vi "Create Timing Diagram from Trigger Position.vi"(11 "Relative Trigger Position in":dbl[](array[numeric])) -> (3 "Timing Diagram":digitalwaveform[](array[waveform]))   [LabVIEW 2024]
uses:
  <vilib>/Waveform/DWDTOps.llb/Digital Pattern Generator (Single Value).vi
  <vilib>/Waveform/DWDTOps.llb/DWDT Append Digital Samples.vi
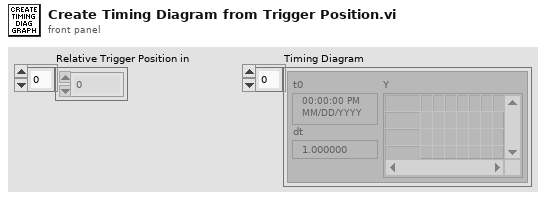
[diagram p1: front panel]
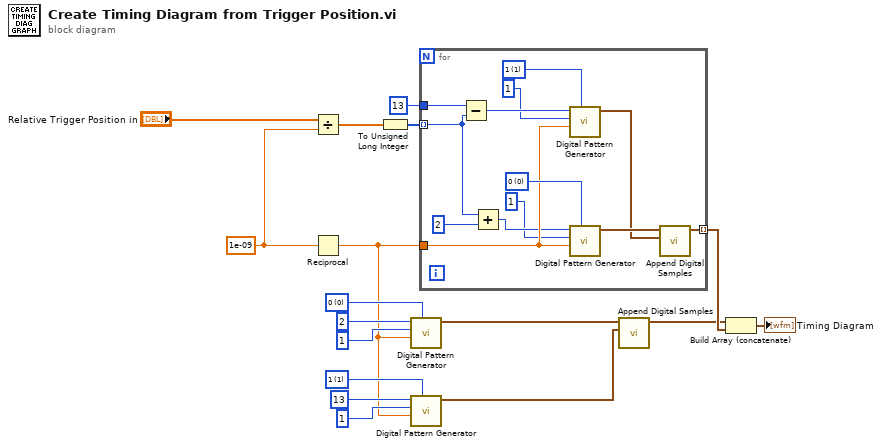
[diagram p0: block diagram]
diagram:
  w7 = u8 1 items=["0", "1", "Z", "L", "H", "X", "T", "V"] ("value")
  w10 = u8 0 items=["0", "1", "Z", "L", "H", "X", "T", "V"] ("value")
  w16 = 1e-09 ("y")
  n1 = Divide(x="Relative Trigger Position in", y=w16) -> (x/y=w2:dbl[])
  n2 = Reciprocal(x=w16) -> (1/x=w1:dbl)
  n3 = To Unsigned Long Integer(number=w2) -> (unsigned 32bit integer=w3:u32[])
  n4 = call-poly <vilib>:"Digital Pattern Generator.vi"("value"=w10, "sample rate"=w1, "number of signals"=u32 1, "number of samples"=u32 2) -> ("digital waveform"=w6:digitalwaveform)  [unwired: 6 in, 1 out]
  n5 = call-poly <vilib>:"Digital Pattern Generator.vi"("value"=w7, "sample rate"=w1, "number of signals"=u32 1, "number of samples"=u32 13) -> ("digital waveform"=w5:digitalwaveform)  [unwired: 6 in, 1 out]
  n6 = for {
    tunnel: w3 -> [w21] mode=indexing
    tunnel: u32 13 -> [w30]
    tunnel: [w26] -> w14 mode=indexing
    tunnel: w1 -> [w25]
    w29 = u8 0 items=["0", "1", "Z", "L", "H", "X", "T", "V"] ("value")
    w28 = u8 1 items=["0", "1", "Z", "L", "H", "X", "T", "V"] ("value")
    n7 = Subtract(x=w30, y=w21) -> (x-y=w20:u32)
    n8 = Add(x=w21, y=u32 2) -> (x+y=w22:u32)
    n9 = call-poly <vilib>:"Digital Pattern Generator.vi"("value"=w28, "sample rate"=w25, "number of signals"=u32 1, "number of samples"=w20) -> ("digital waveform"=w23:digitalwaveform)  [unwired: 6 in, 1 out]
    n10 = call-poly <vilib>:"Digital Pattern Generator.vi"("value"=w29, "sample rate"=w25, "number of signals"=u32 1, "number of samples"=w22) -> ("digital waveform"=w24:digitalwaveform)  [unwired: 6 in, 1 out]
    n11 = call-poly <vilib>:"Append Digital Samples.vi"("digital waveform B"=w23, "digital waveform A"=w24) -> ("digital waveform out"=w26:digitalwaveform)  [unwired: 8 in, 1 out]
  }
  n12 = call-poly <vilib>:"Append Digital Samples.vi"("digital waveform B"=w5, "digital waveform A"=w6) -> ("digital waveform out"=w13:digitalwaveform)  [unwired: 8 in, 1 out]
  n13 = Build Array (concatenate)(w13, w14) -> (→"Timing Diagram":digitalwaveform[])
